vi "Hardware Out - VRHall-1.vi"(11 "FPGA Ref":T1) -> ()   [LabVIEW 2015, in "ECS-RT.lvlib"]
uses:
  ECS-RT.lvlib
  Typedefs/FPGA Refs/Generic FPGA Ref.ctl
  <vilib>/Utility/error.llb/Error Cluster From Error Code.vi
  <vilib>/rvi/errors/niLvFpgaAdjustHostInterfaceError.vi
  <vilib>/rvi/interface/nirviReadWriteControl/nirviReadWriteControl.xnode
  <vilib>/rvi/interface/Simulation/niFpgaSimulationCallBeginRW.vi
  NiFpgaLv.dll
  ECS-Shared.lvlib
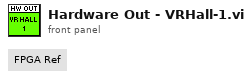
[diagram p1: front panel]
types:
  T1 = typedef "ECS-Shared.lvlib/Generic FPGA Ref.ctl" = refnum<k20>
  T2 = cluster{"Boolean array[0]":bool, "Boolean array[1]":bool, "Boolean array[2]":bool, "Boolean array[3]":bool, "Boolean array[4]":bool, "Boolean array[5]":bool}
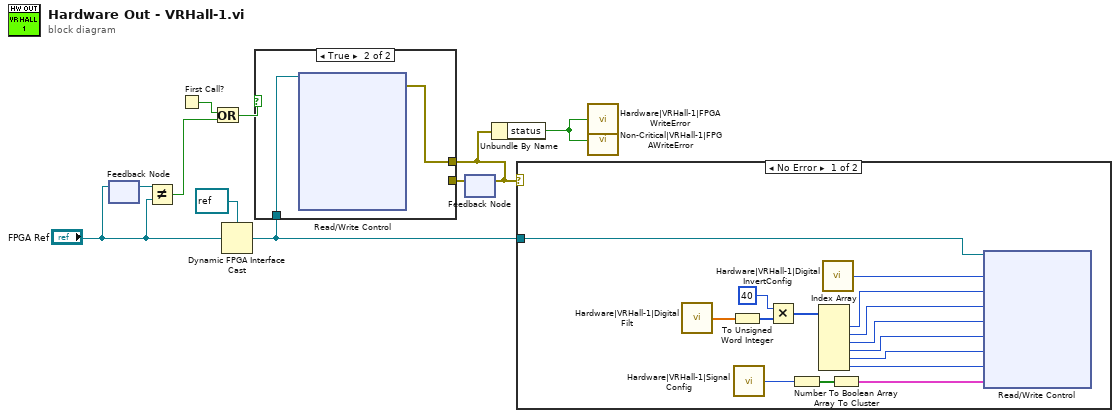
[diagram p0: block diagram]
diagram:
  n1 = feedback #1() -> (w6:T1)  [unwired: 1 in]
  n2 = feedback-in #1("FPGA Ref") -> ()
  n3 = Not Equal?(x=w6, y="FPGA Ref") -> (x != y?=w5:bool)
  n4 = First Call?() -> (First Call?: T/F=w7:bool)
  n5 = Or(x=w7, y=w5) -> (x .or. y?=w8:bool)
  n6 = Dynamic FPGA Interface Cast(Session In=refnum<k20> refnum ("NI 9411"), Type="FPGA Ref") -> (Session Out=w3:refnum<k20>)
  n7 = feedback #2() -> (w9:errorcluster)  [unwired: 1 in]
  n8 = case shown="True" w8 {
    tunnel: [w11 w12] -> w2
    tunnel: w9 -> [w11 _]
    tunnel: w3 -> [_ w13]
    frame False {
    }
    frame True {
      n9 = xnode "Read/Write Control"("FPGA VI Reference In"=w13) -> ("error out"=w12:errorcluster)  [unwired: 9 in, 1 out]
    }
  }
  n10 = feedback-in #2(w2) -> ()
  n11 = Unbundle By Name(w2) -> ("status"=w1:bool)
  n12 = case shown="No Error" w2 {
    tunnel: w3 -> [w24 _]
    frame No Error {
      n13 = call "Hardware|VRHall-1|DigitalFilt"() -> ("Value"=w28:sgl[])
      n14 = To Unsigned Word Integer(number=w28) -> (unsigned 16bit integer=w27:u16[])
      n15 = call "Hardware|VRHall-1|SignalConfig"() -> ("Value"=w16:u32)
      n16 = Multiply(x=u16 40 ("y"), y=w27) -> (x*y=w26:u16[])
      n17 = Number To Boolean Array(number=w16) -> (Boolean array=w15:bool[])
      n18 = Index Array(array=w26) -> (element #1=w22:u16, element #2=w21:u16, element #3=w20:u16, element #4=w19:u16, element #5=w18:u16, element #6=w17:u16)  [unwired: 6 in]
      n19 = call "Hardware|VRHall-1|DigitalInvertConfig"() -> ("Value"=w23:u32)
      n20 = Array To Cluster(array=w15) -> (cluster=w14:T2)
      n21 = xnode "Read/Write Control"("FPGA VI Reference In"=w24, "VRHall-1.Invert"=w23, "VRHall-1.1.Filt"=w22, "VRHall-1.2.Filt"=w21, "VRHall-1.3.Filt"=w20, "VRHall-1.4.Filt"=w19, "VRHall-1.5.Filt"=w18, "VRHall-1.6.Filt"=w17, "VRHall-1.Control"=w14) -> ()  [unwired: 1 in, 2 out]
    }
    frame Error {
    }
  }
  n22 = call "Hardware|VRHall-1|FPGAWriteError"("Value"=w1) -> ()
  n23 = call "Non-Critical|VRHall-1|FPGAWriteError"("Fault"=w1) -> ()  [unwired: 2 in]
